vi "dev_make-gaussian.vi"(9 "StdDev":dbl, 10 "Mean":dbl, 11 "in":dbl format="%#_13g") -> (3 "out":dbl)   [LabVIEW 2024]
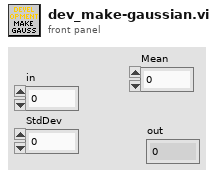
[diagram p1: front panel]
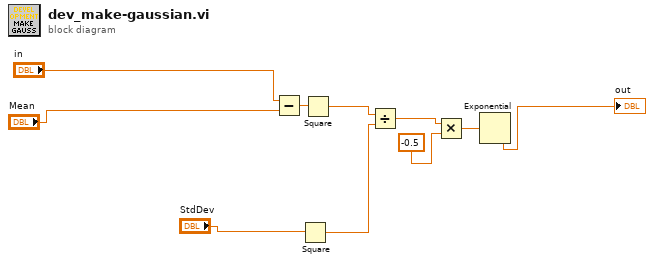
[diagram p0: block diagram]
diagram:
  n1 = Subtract(x="in", y="Mean") -> (x-y=w3:dbl)
  n2 = Square(x="StdDev") -> (x^2=w5:dbl)
  n3 = Square(x=w3) -> (x^2=w4:dbl)
  n4 = Divide(x=w4, y=w5) -> (x/y=w6:dbl)
  n5 = Multiply(x=w6, y=-0.5) -> (x*y=w8:dbl)
  n6 = Exponential(1:w8) -> (0:→"out":dbl)
